vi "emi_Set System ID.vi"(7 "System ID(0)":u8, 9 "error in (no error)":errorcluster) -> (10 "error out":errorcluster)   [LabVIEW 2011]
doc: "Checks wheter the application id closeing,"
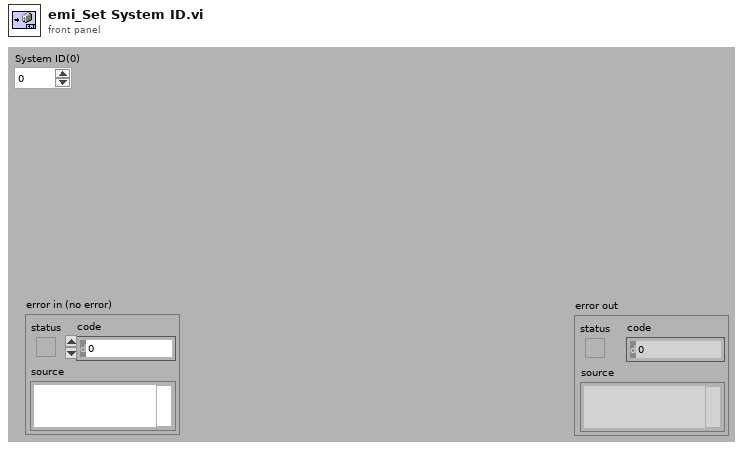
[diagram p1: front panel]
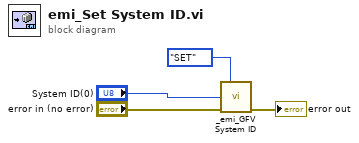
[diagram p0: block diagram]
diagram:
  n1 = call "_emi_GFV System ID.vi"("Action(GET)"=enum16{"GET", "SET"}."SET", "System ID in"="System ID(0)", "error in (no error)"="error in (no error)") -> ("error out"=→"error out":errorcluster)  [unwired: 11 in, 1 out]
